vi "Query Burst.vi"(8 "error in (no error)":errorcluster, 10 "Channel (0: Channel 1)":T1 items=["Channel 1", "Channel 2"], 11 "VISA resource name":refnum<visa-resource-name>) -> (0 "error out":errorcluster, 1 "Burst Mode":u16(ring)=1 items=["Triggered", "Gated"], 2 "Burst Enabled?":bool=TRUE, 3 "VISA resource name out":refnum<visa-resource-name>, 4 "Burst Count":i32=5)   [LabVIEW 2015, in "Tektronix AFG 3000 Series.lvlib"]
uses:
  Tektronix AFG 3000 Series.lvlib
  controls.llb/Channel.ctl
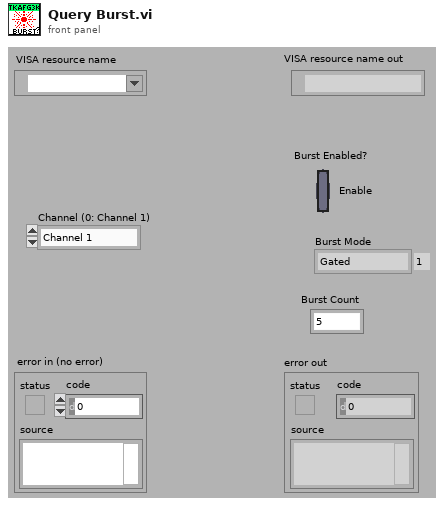
[diagram p1: front panel]
types:
  T1 = typedef "Channel.ctl" = u16
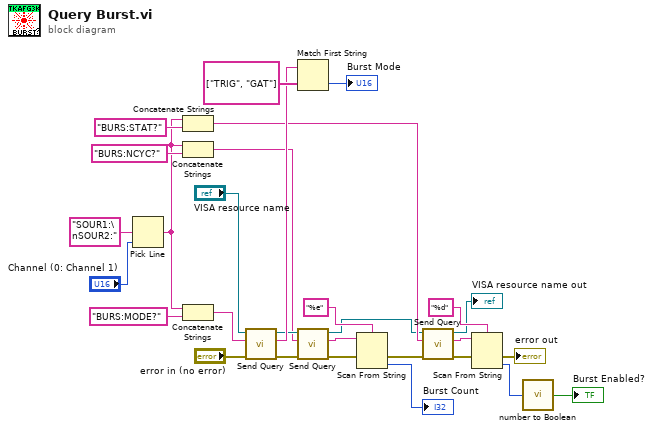
[diagram p0: block diagram]
diagram:
  n1 = Pick Line(multi-line string="SOUR1:\nSOUR2:" ("string (\"\")"), line index="Channel (0: Channel 1)") -> (output string=w12:string)  [unwired: 1 out]
  n2 = Concatenate Strings(w12, "BURS:STAT?" ("format string")) -> (w11:string)
  n3 = Concatenate Strings(w12, "BURS:NCYC?" ("format string")) -> (w17:string)
  n4 = Concatenate Strings(w12, "BURS:MODE?" ("format string")) -> (w24:string)
  n5 = call "Send Query.vi"("error in (no error)"="error in (no error)", "write buffer"=w24, "VISA resource name"="VISA resource name") -> ("error out"=w16:errorcluster, "read buffer"=w23:string, "VISA resource name out"=w18:refnum<visa-resource-name>)  [unwired: 1 in, 5 out]
  n6 = Match First String(2:string[] ["TRIG", "GAT"] ("string array"), 3:w23) -> (0:→"Burst Mode":i32)  [unwired: 1 out]
  n7 = call "Send Query.vi"("error in (no error)"=w16, "write buffer"=w17, "VISA resource name"=w18) -> ("error out"=w9:errorcluster, "read buffer"=w15:string, "VISA resource name out"=w10:refnum<visa-resource-name>)  [unwired: 1 in, 5 out]
  n8 = Scan From String(format string="%e", input string=w15, error in=w9) -> (error out=w8:errorcluster, output 1=→"Burst Count":i32)  [unwired: 1 in, 3 out]
  n9 = call "Send Query.vi"("error in (no error)"=w8, "write buffer"=w11, "VISA resource name"=w10) -> ("error out"=w4:errorcluster, "read buffer"=w6:string, "VISA resource name out"=→"VISA resource name out":refnum<visa-resource-name>)  [unwired: 1 in, 5 out]
  n10 = Scan From String(format string="%d", input string=w6, error in=w4) -> (error out=→"error out":errorcluster, output 1=w5:i32)  [unwired: 1 in, 3 out]
  n11 = call "number to Boolean.vi"("Numeric"=w5) -> ("Boolean"=→"Burst Enabled?":bool)
